vi "运维调试_CODCr.vi"() -> ()   [LabVIEW 2016, in "CODCr库.lvlib"]
uses:
  <vilib>/Utility/miscctls.llb/LVPointTypeDef.ctl
  <vilib>/ptbypt/NI_PtbyPt.lvlib
  <vilib>/Utility/config.llb/NI_LVConfig.lvlib
panel:
  in  "MB通信方式选择":enum16{"串口", "TCP"}(ring)
  in  "释放串口":bool
  in  "打开串口":bool
  in  "加标回收测试":bool
  in  "平行样测试":bool
  in  "定时启动":bool
  out "COM口":string
  in  "空白测试":bool
  in  "隐藏按钮":bool
  in  "写入消解温度时长":bool
  in  "保存KB值":bool
  in  "标样核查":bool
  out "启动时间":timestamp format="%<%Y/%m/%d %H:%M:%S>T"
  out "主循环次数":i32
  out "status":bool
  out "启动测量模式":T1(ring)
  out "曲线斜率B":sgl format="%#_10g"
  out "曲线斜率K":sgl format="%#_10g"
  out "量程上限":sgl
  out "量程下限":sgl
  out "消解时长":u16
  out "消解温度":u16
  out "测量精度":u16
  out "测量结果":sgl
  out "标样参考值":sgl
  out "量程":u16
  out "工作状态":T1(ring)
  out "仪器时间":timestamp format="%<%X\n%x>T"
  out "关键参数区":T2
  out "状态告警区":T3
  out "测量数据区":T4 {"单位" items=["ug/L", "mg/L", "ppm", "mg/m3", "cm", "ppb", "ug/m3", "%", "nmol/mol", "umol/mol", "MPN/L", "MPN/100ml", "ng/m3", "NTU", "无量纲", "ms/cm", "us/cm", "℃", "mV", "万个/L"]}
  out "系统时间":timestamp format="%<%Y/%m/%d %H:%M:%S>T"
  in  "停止":bool
  in  "校时":bool
  in  "标样校准":bool
  in  "空白校准":bool
  in  "零点核查":bool
  in  "跨度核查":bool
  in  "水样测试":bool
  in  "返回":bool
  in  "设置":bool
  # "mg/L"
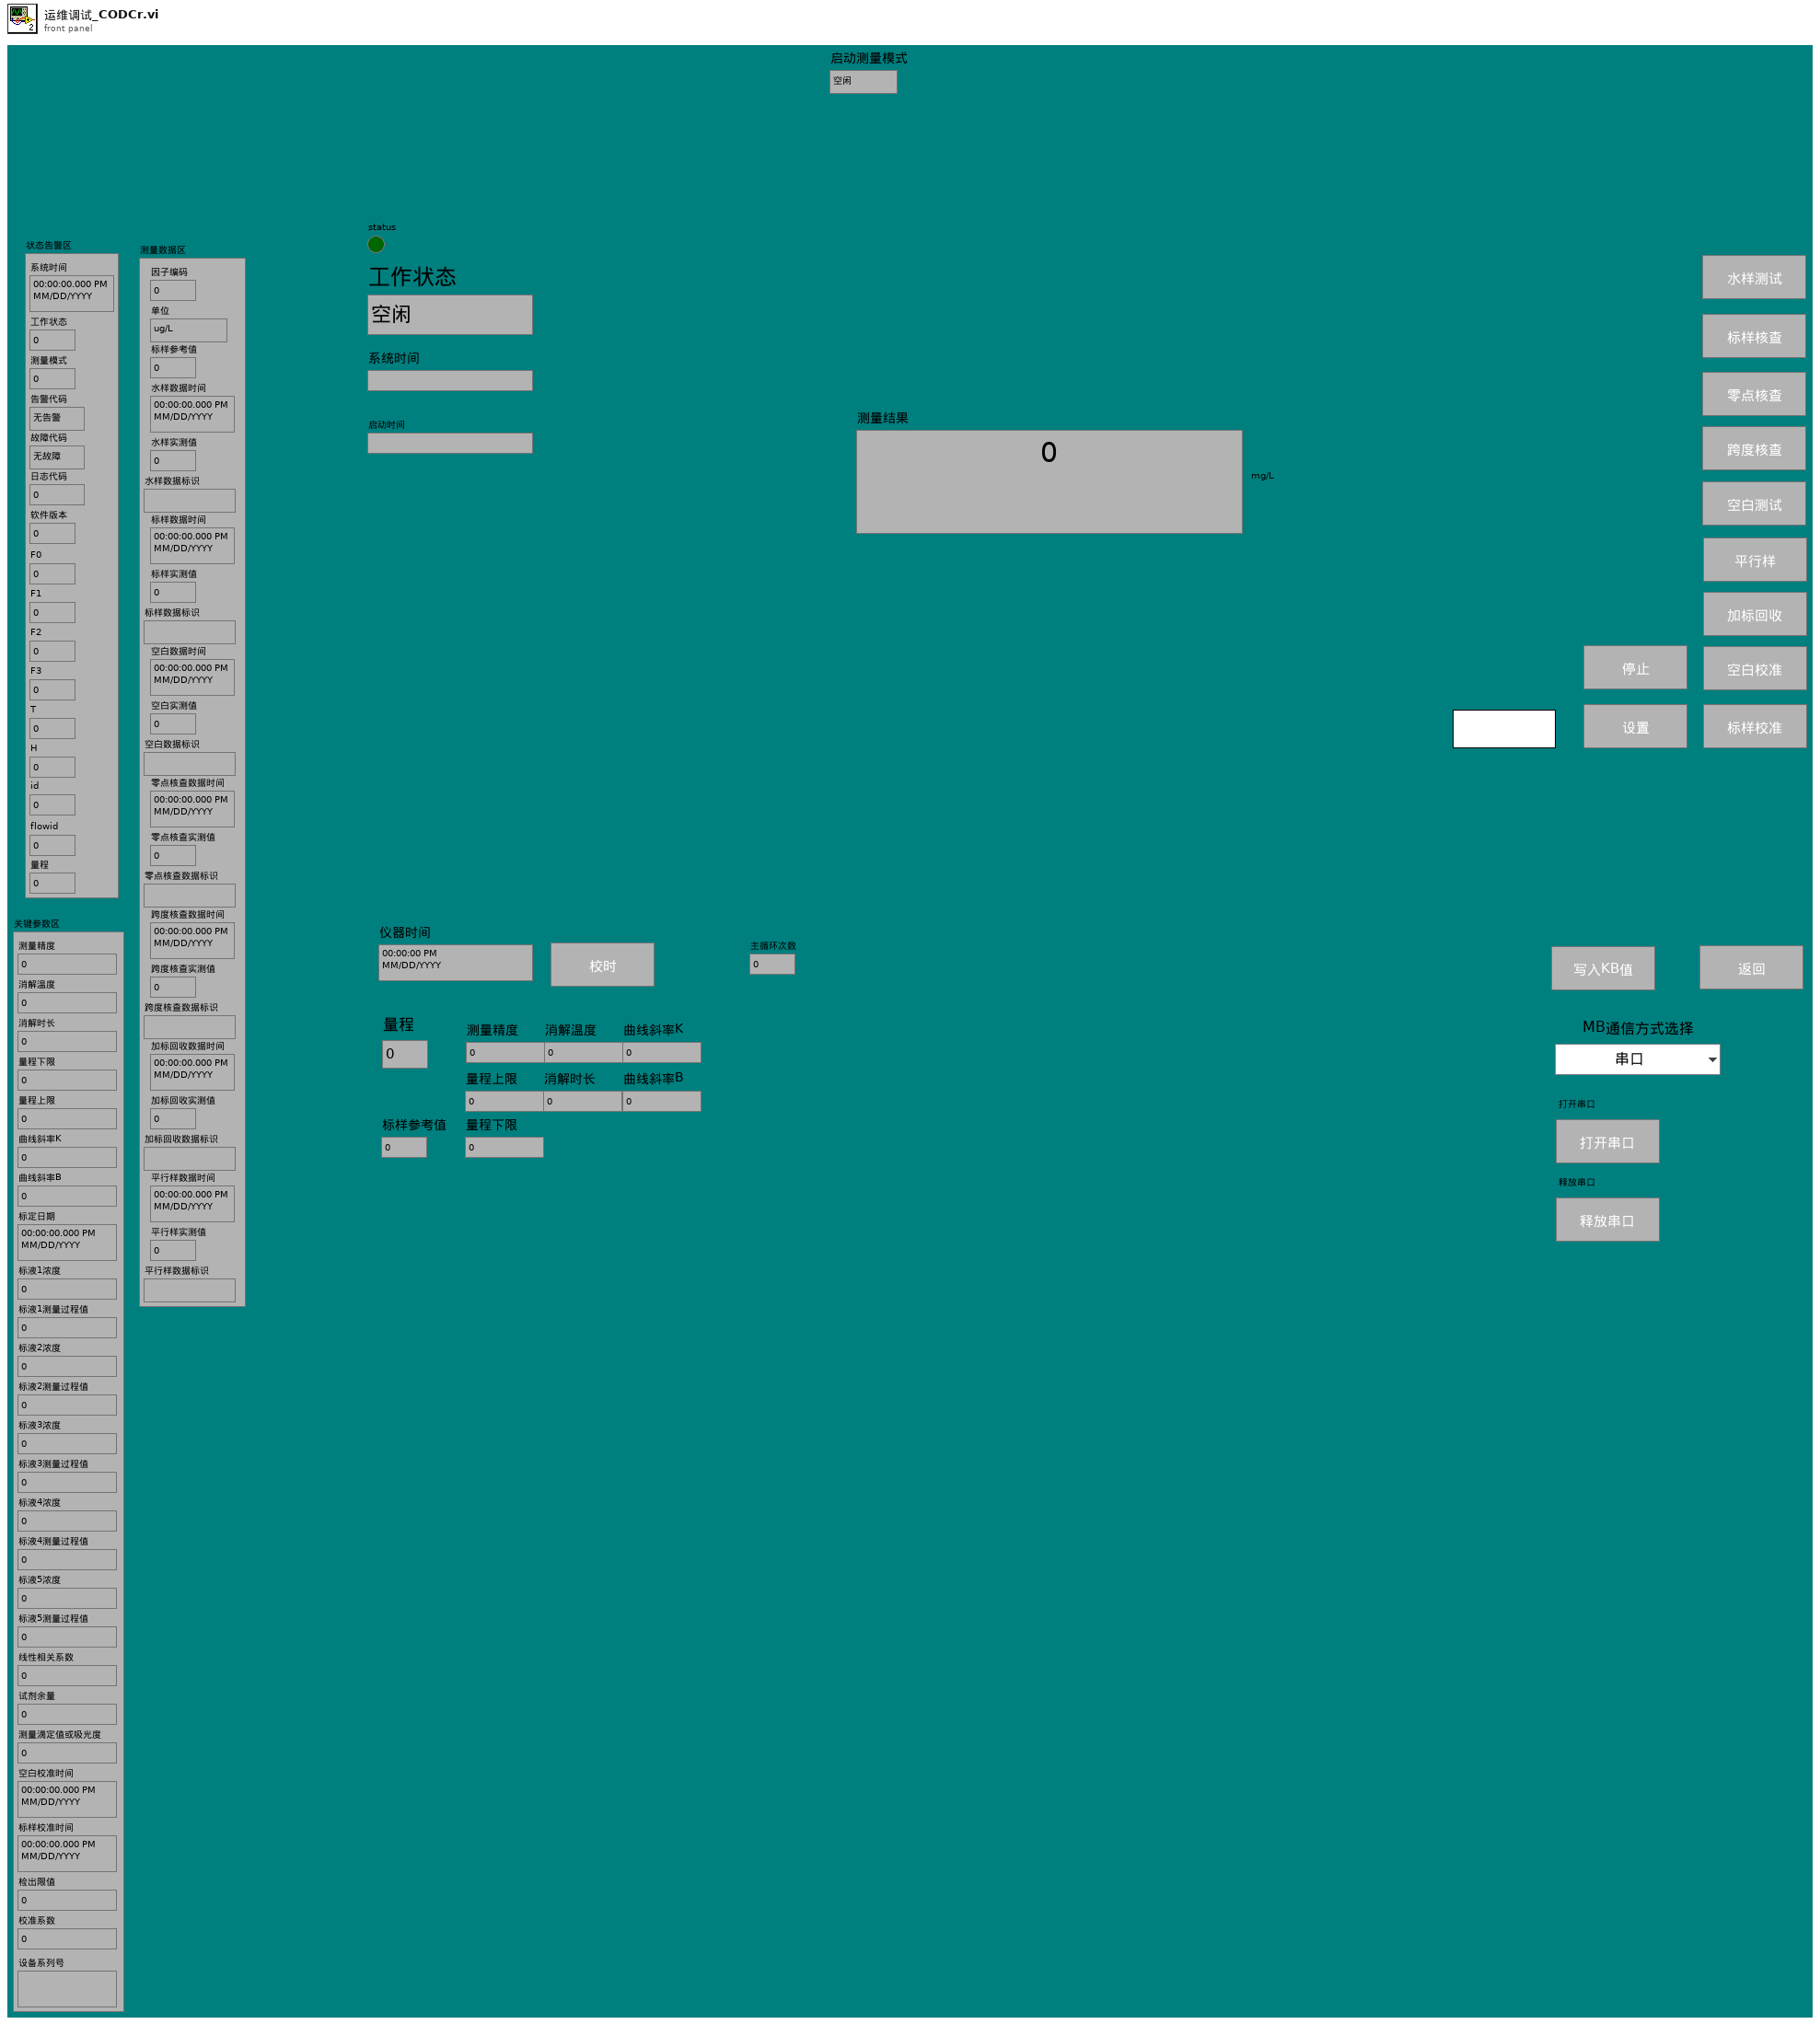
[diagram p1: front panel]
types:
  T1 = enum16{"空闲", "水样测试", "标样核查", "零点核查", "跨度核查", "空白测试", "平行样测试", "加标回收", "空白校准", "标样校准", "初始化（清洗）"}
  T2 = cluster{"测量精度":u16, "消解温度":u16, "消解时长":u16, "量程下限":sgl, "量程上限":sgl, "曲线斜率K":sgl, "曲线斜率B":sgl, "标定日期":timestamp, "标液1浓度":sgl, "标液1测量过程值":sgl, "标液2浓度":sgl, "标液2测量过程值":sgl, "标液3浓度":sgl, "标液3测量过程值":sgl, "标液4浓度":sgl, "标液4测量过程值":sgl, "标液5浓度":sgl, "标液5测量过程值":sgl, "线性相关系数":sgl, "试剂余量":u32, "测量滴定值或吸光度":sgl, "空白校准时间":timestamp, "标样校准时间":timestamp, "检出限值":sgl, "校准系数":sgl, "设备系列号":string}
  T3 = cluster{"系统时间":timestamp, "工作状态":u16, "测量模式":u16, "告警代码":enum16{"无告警", "缺试剂告警", "缺水样告警", "缺蒸馏水告警", "缺标液告警", "仪表漏液告警", "标定异常告警", "超量程告警", "加热异常", "低试剂预警", "超上限告警", "超下限告警", "仪表内部其他异常", "滴定异常告警", "电极异常告警", "量程切换告警", "参数设置告警", "PH电极电位异常", "电导率电极异常", "浊度光度异常", "溶解氧电极异常", "溶解氧光强异常", "温度异常告警", "PH异常告警", "溶解氧异常告警", "电导率异常告警", "浊度异常告警", "叶绿素异常告警", "藻密度异常告警", "蓝绿藻异常告警", "ORP异常告警", "氨氮异常告警", "清洁刷异常告警", "SD卡异常告警", "蓝牙异常告警", "Wifi异常告警", "流程异常告警"}, "故障代码":enum16{"无故障", "电机故障", "温度故障", "通讯故障", "滴定故障"}, "日志代码":u16, "软件版本":u16, "F0":sgl, "F1":sgl, "F2":sgl, "F3":sgl, "T":sgl, "H":sgl, "id":u16, "flowid":u16, "量程":u16}
  T4 = cluster{"因子编码":u32, "单位":u16, "标样参考值":sgl, "水样数据时间":timestamp, "水样实测值":sgl, "水样数据标识":string, "标样数据时间":timestamp, "标样实测值":sgl, "标样数据标识":string, "空白数据时间":timestamp, "空白实测值":sgl, "空白数据标识":string, "零点核查数据时间":timestamp, "零点核查实测值":sgl, "零点核查数据标识":string, "跨度核查数据时间":timestamp, "跨度核查实测值":sgl, "跨度核查数据标识":string, "加标回收数据时间":timestamp, "加标回收实测值":sgl, "加标回收数据标识":string, "平行样数据时间":timestamp, "平行样实测值":sgl, "平行样数据标识":string}
  T5 = cluster{"命令":string, "测量模式":enum16{"水样测量", "标样核查", "零点核查", "跨度核查", "空白测试", "加标回收", "平行样", "校零", "校标"}, "CODCr量程切换":enum32{"H", "L", "AUTO"}}
  T6 = cluster{"测量模式":enum16{"水样测量", "标样核查", "零点核查", "跨度核查", "空白测试", "加标回收", "平行样", "校零", "校标"}}
  T7 = cluster{"仪器测试类型":enum16{"水样测试", "标样核查", "空白测试", "跨度核查"}, "周期设置类型":enum16{"定点启动", "间隔启动"}, "定时功能启用":bool, "定时间隔":dbl, "24H周期设置":bool[]}
  T8 = typedef "LVDateTimeRec.ctl" = cluster{"秒数的小数部分":dbl, "秒":i32, "分":i32, "时":i32, "日":i32, "月":i32, "年":i32, "天数（周）":i32, "天数（年）":i32, "DST":i32}
  T9 = typedef "LVPointTypeDef.ctl" = cluster{"Horizontal":i16, "Vertical":i16}
  T10 = typedef "NI_LVConfig.lvlib/Config Data RefNum.ctl" = refnum<k1>
  T11 = cluster{"运行模式":enum16{"维护模式", "常规模式", "应急模式", "质控模式"}}
  T12 = cluster{"时间标识":timestamp, "监测值":sgl, "单位":u16, "数据标识":string, "因子编码":u32, "标样参考值":sgl, "F0":sgl, "F1":sgl, "F2":sgl, "F3":sgl, "温度":sgl, "湿度":sgl, "量程标识":string}
  T13 = cluster{"时间标识":timestamp, "设备":string, "日志信息":string}
  T14 = cluster{"时间标识":timestamp, "参数":string, "日志信息":string, "流程参数":string}
  T15 = enum16{"无告警", "缺试剂告警", "缺水样告警", "缺蒸馏水告警", "缺标液告警", "仪表漏液告警", "标定异常告警", "超量程告警", "加热异常", "低试剂预警", "超上限告警", "超下限告警", "仪表内部其他异常", "滴定异常告警", "电极异常告警", "量程切换告警", "参数设置告警", "PH电极电位异常", "电导率电极异常", "浊度光度异常", "溶解氧电极异常", "溶解氧光强异常", "温度异常告警", "PH异常告警", "溶解氧异常告警", "电导率异常告警", "浊度异常告警", "叶绿素异常告警", "藻密度异常告警", "蓝绿藻异常告警", "ORP异常告警", "氨氮异常告警", "清洁刷异常告警", "SD卡异常告警", "蓝牙异常告警", "Wifi异常告警", "流程异常告警"}
  T16 = cluster{"时间标识":timestamp, "设备":string, "日志信息":string, "流程参数":string}
  T17 = enum16{"水样测量", "标样核查", "零点核查", "跨度核查", "空白测试", "加标回收", "平行样", "校零", "校标"}
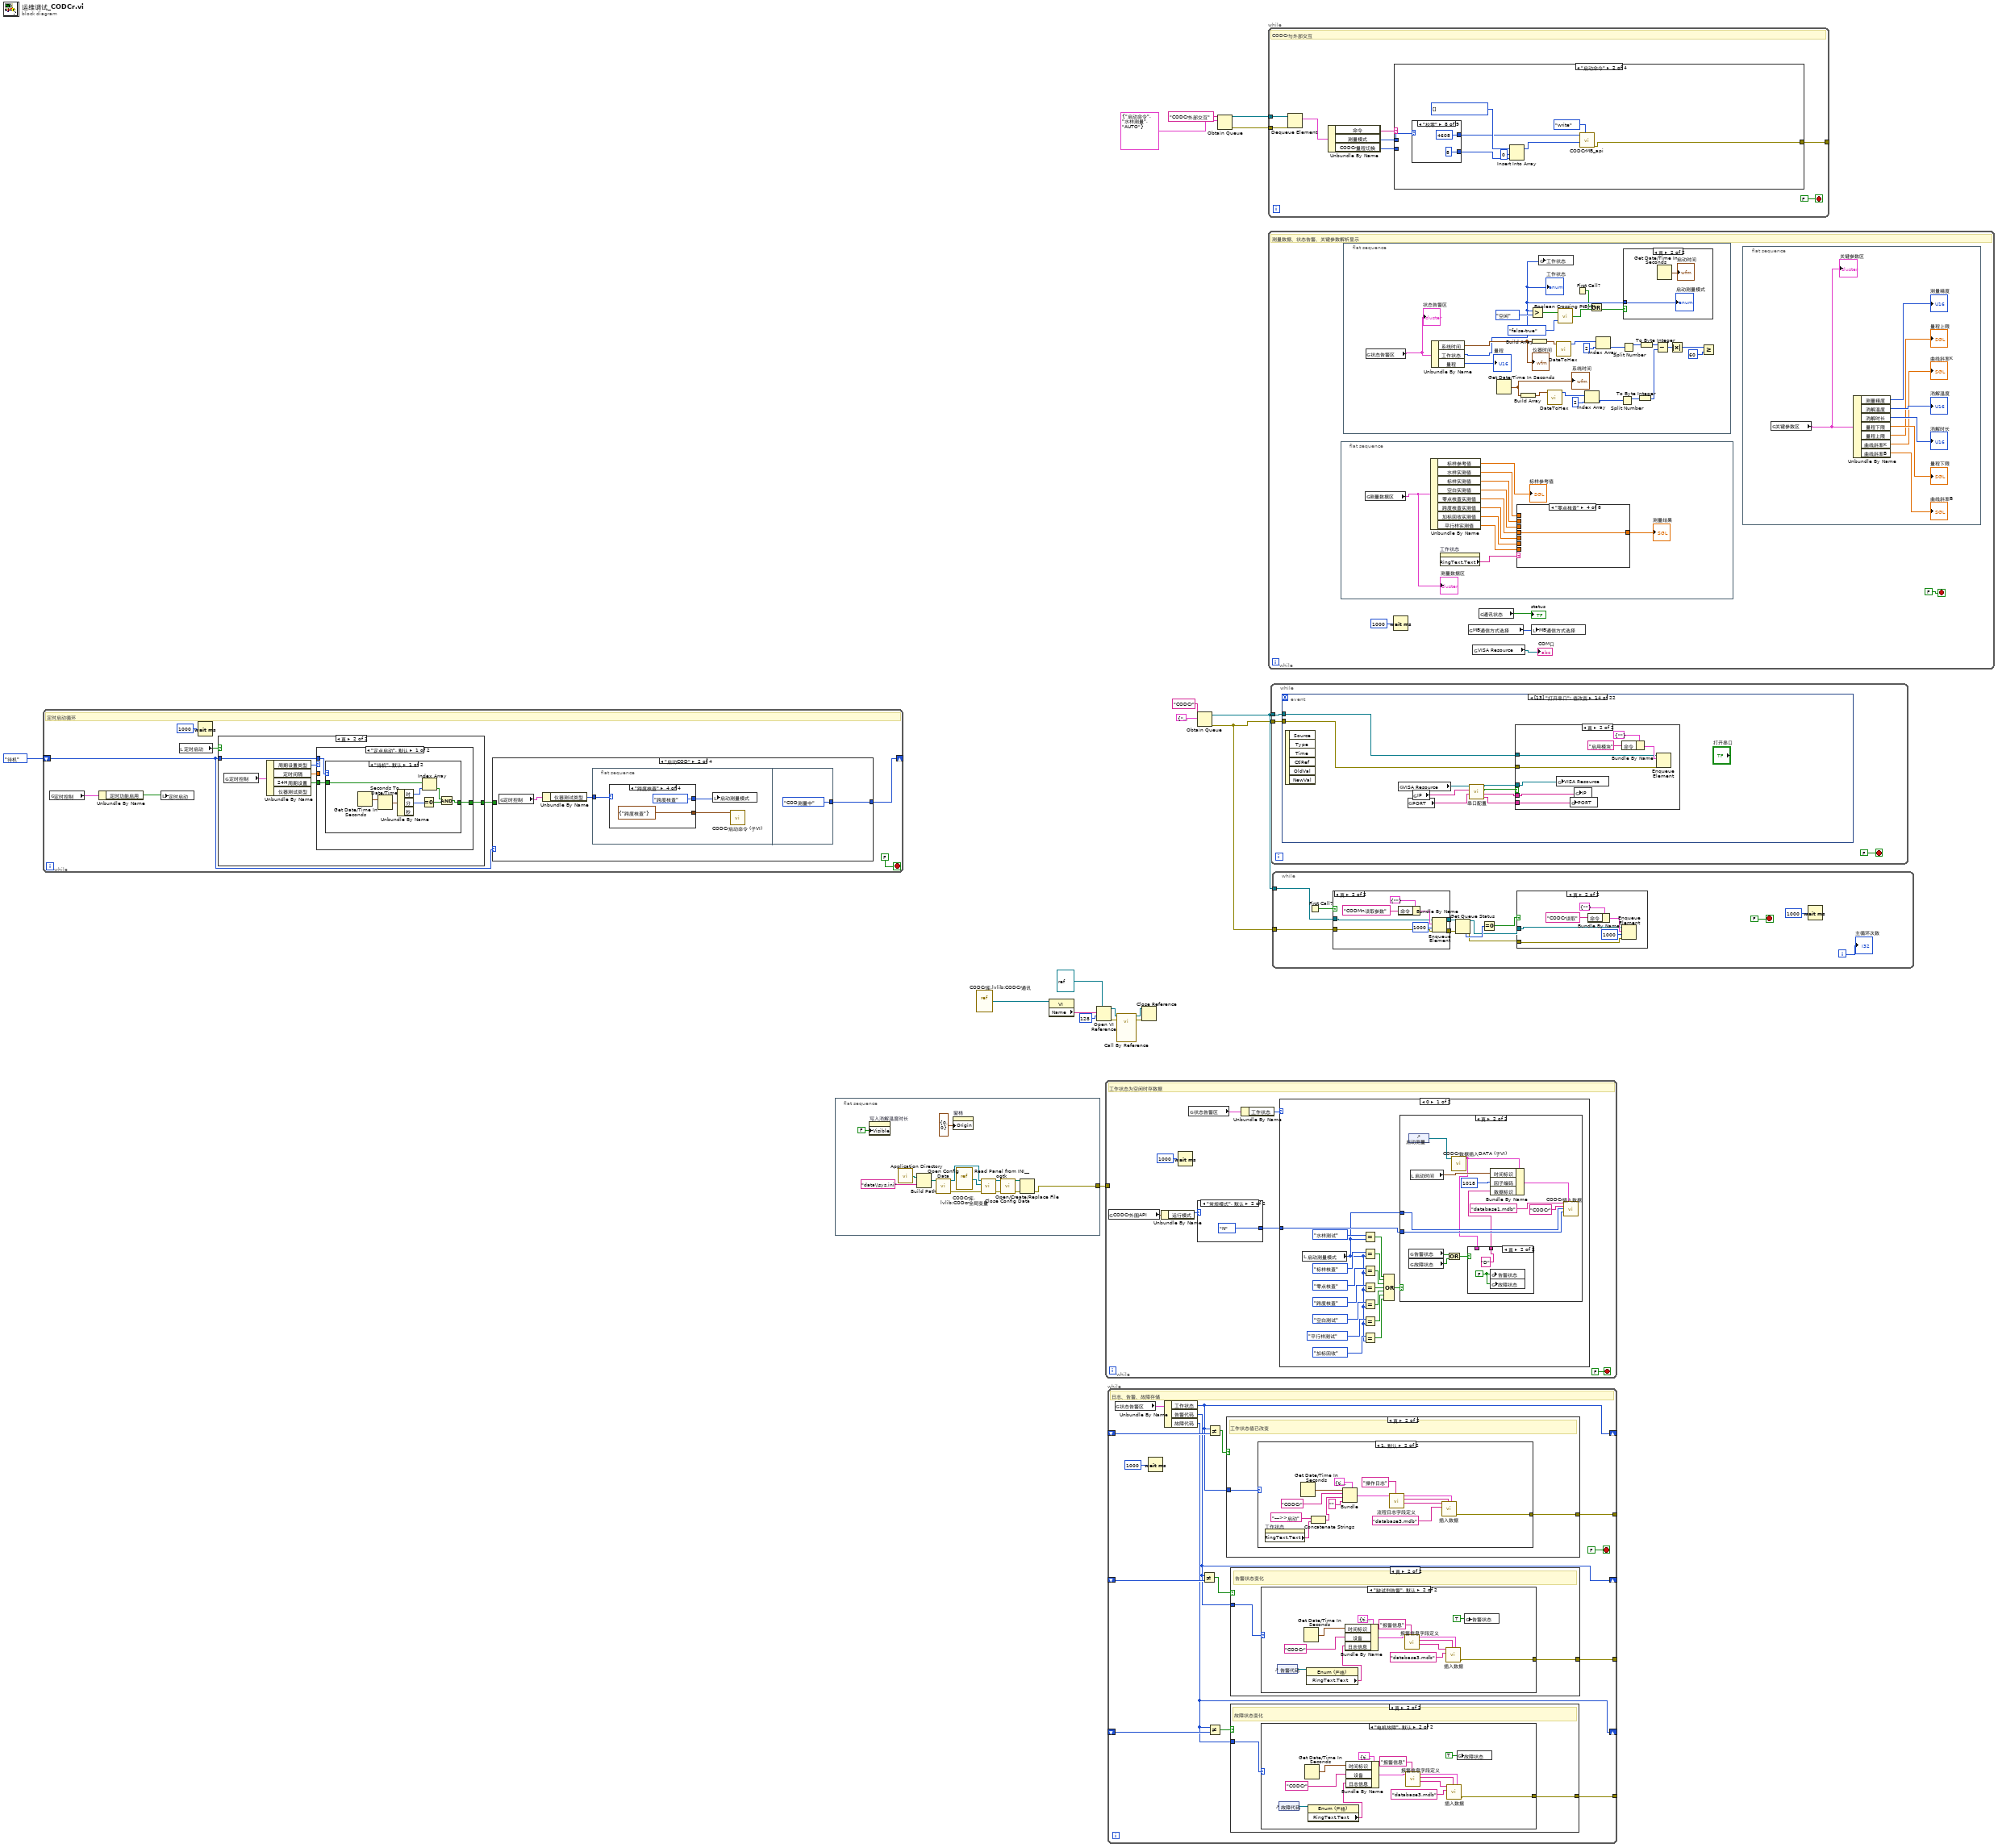
[diagram p0: block diagram]
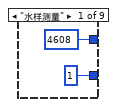
[diagram p5: hidden frame]
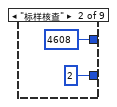
[diagram p6: hidden frame]
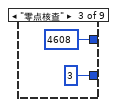
[diagram p7: hidden frame]
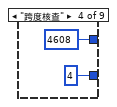
[diagram p8: hidden frame]
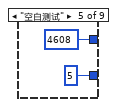
[diagram p9: hidden frame]
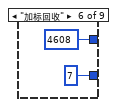
[diagram p10: hidden frame]
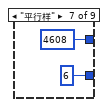
[diagram p11: hidden frame]
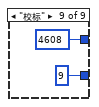
[diagram p12: hidden frame]
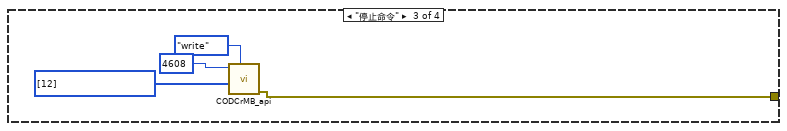
[diagram p13: hidden frame]
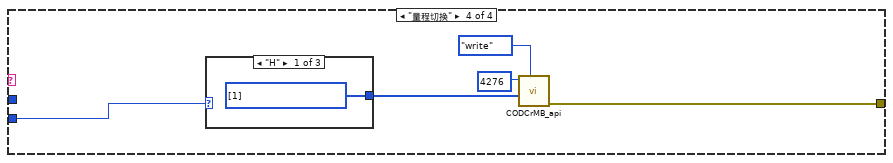
[diagram p14: hidden frame]
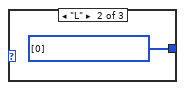
[diagram p15: hidden frame]
diagram:
  n1 = while {
    shift-right: [w24] -> _
    shift-left: enum16{"待机", "启动COD", "COD测量中", "延时"}."待机" -> [w23]
    stop <- FALSE stop-if-true
    # "定时启动循环"
    n2 = global read "CODcr全局变量.vi" "定时控制"() -> (w20:T7)
    n3 = Unbundle By Name(w20) -> ("定时功能启用"=w19:bool)
    n4 = local write "定时启动"(w19) -> ()
    n5 = local read "定时启动"() -> (w21:bool)
    n6 = Wait (ms)(milliseconds to wait=u32 1000 ("等待时间（毫秒）")) -> ()  [unwired: 1 out]
    n7 = case shown="真" w21 {
      tunnel: w23 -> [_ w59]
      tunnel: [_ w58] -> w22
      frame False {
      }
      frame True {
        n8 = global read "CODcr全局变量.vi" "定时控制"() -> (w57:T7)
        n9 = Unbundle By Name(w57) -> ("周期设置类型"=w60:enum16{"定点启动", "间隔启动"}, "定时间隔"=w61:dbl, "24H周期设置"=w62:bool[])  [unwired: 1 out]
        n10 = case shown="\"定点启动\", 默认" w60 {
          tunnel: w61 -> [_ w77]
          tunnel: w62 -> [w65 _]
          tunnel: w59 -> [w63 w80]
          tunnel: [w64 w75] -> w58
          frame "定点启动", Default {
            n11 = case shown="\"待机\", 默认" w63 {
              tunnel: w65 -> [w71 _]
              tunnel: [w66 _] -> w64
              frame "待机", Default {
                n12 = Get Date/Time In Seconds() -> (seconds since 1Jan1904=w73:timestamp)
                n13 = Seconds To Date/Time(time stamp (now)=w73) -> (date time rec=w72:T8)  [unwired: 1 in]
                n14 = Unbundle By Name(w72) -> ("时"=w70:i32, "分"=w69:i32)  [unwired: 1 out]
                n15 = Equal To 0?(x=w69) -> (x = 0?=w67:bool)
                n16 = Index Array(array=w71, index=w70) -> (element=w68:bool)
                n17 = Compound Arithmetic op=AND ("复合运算")(w68, w67) -> (w66:bool)
              }
              frame "启动COD" {
              }
            }
          }
          frame "间隔启动" {
            n18 = Multiply(x=w77, y=60.0) -> (x*y=w74:dbl)
            n19 = feedback #1(w74) -> (w79:dbl)
            n20 = case shown="\"待机\"" w80 {
              tunnel: w79 -> [_ w82]
              tunnel: [_ w81] -> w78
              frame Default {
              }
              frame "待机" {
                n21 = Increment(x=w82) -> (x+1=w81:dbl)
              }
            }
            n22 = feedback-in #1(w78) -> ()
            n23 = Greater Or Equal?(x=w78, y=w74) -> (x >= y?=w75:bool)
          }
        }
      }
    }
    n24 = case shown="\"启动COD\"" w23 {
      tunnel: [w27 w33 w47 enum16{"待机", "启动COD", "COD测量中", "延时"}."待机"] -> w24
      tunnel: w22 -> [w30 _ _ _]
      frame "待机", Default {
        n25 = Select(t=enum16{"待机", "启动COD", "COD测量中", "延时"}."启动COD", s=w30, f=enum16{"待机", "启动COD", "COD测量中", "延时"}."待机") -> (s? t:f=w27:enum16{"待机", "启动COD", "COD测量中", "延时"})
      }
      frame "启动COD" {
        n26 = global read "CODcr全局变量.vi" "定时控制"() -> (w31:T7)
        n27 = Unbundle By Name(w31) -> ("仪器测试类型"=w32:enum16{"水样测试", "标样核查", "空白测试", "跨度核查"})
        n28 = flat-sequence {
          tunnel: w32 -> [w36]
          tunnel: [enum16{"待机", "启动COD", "COD测量中", "延时"}."COD测量中"] -> w33
          frame #0 {
            n29 = case shown="\"跨度核查\"" w36 {
              tunnel: [T6 {"测量模式"=enum."水样测量"} ("启动测量模式") T6 {"测量模式"=enum."标样核查"} ("启动测量模式") T6 {"测量模式"=enum."空白测试"} ("启动测量模式") T6 {"测量模式"=enum."跨度核查"} ("启动测量模式")] -> w35
              tunnel: [T1."水样测试" ("启动测量模式") T1."标样核查" ("启动测量模式") T1."空白测试" ("启动测量模式") T1."跨度核查" ("启动测量模式")] -> w34
              frame "水样测试", Default {
              }
              frame "标样核查" {
              }
              frame "空白测试" {
              }
              frame "跨度核查" {
              }
            }
            n30 = local write "启动测量模式"(w34) -> ()
            n31 = call "CODCr启动命令 (子VI).vi"("启动测量模式"=w35) -> ()  [unwired: 11 in]
          }
          frame #1 {
          }
        }
      }
      frame "COD测量中" {
        n32 = flat-sequence {
          tunnel: [w51] -> w46
          tunnel: [w55] -> w47
          tunnel: w46 -> [w55]
          frame #0 {
            n33 = local read "状态告警区"() -> (w50:T3)
            n34 = Unbundle By Name(w50) -> ("工作状态"=w49:u16)
            n35 = Equal To 0?(x=w49) -> (x = 0?=w48:bool)
            n36 = Select(t=enum16{"待机", "启动COD", "COD测量中", "延时"}."延时", s=w48, f=enum16{"待机", "启动COD", "COD测量中", "延时"}."COD测量中") -> (s? t:f=w51:enum16{"待机", "启动COD", "COD测量中", "延时"})
          }
          frame #1 {
            n37 = Wait (ms)(milliseconds to wait=u32 5000 ("等待时间（毫秒）")) -> ()  [unwired: 1 out]
          }
        }
      }
      frame "延时" {
      }
    }
  }
  n38 = flat-sequence {
    tunnel: [w83] -> w17
    frame #0 {
      n39 = property on="写入消解温度时长" class="Bool"("Visible"=FALSE ("可见")) -> ()  [unwired: 2 in, 2 out]
      n40 = call <vilib>:"Application Directory.vi"() -> ("Application Directory"=w93:path)
      n41 = Build Path(base path=w93, name or relative path="data\\sys.ini" ("名称或相对路径")) -> (appended path=w91:path)
      n42 = call <vilib>:"Open Config Data.vi"("configuration file path"=w91) -> ("error out"=w87:errorcluster, "refnum"=w90:T10)  [unwired: 8 in, 1 out]
      n43 = property on="窗格" class="Pane"("Origin"=T9 {"Horizontal"=0, "Vertical"=0} ("原点")) -> ()  [unwired: 2 in, 2 out]
      n44 = vi-ref "CODCr库.lvlib:CODcr全局变量.vi"() -> (w89:refnum<vi>)
      n45 = call <userlib>:"Read Panel from INI__ogtk.vi"("error in (no error)"=w87, "VI ref"=w89, "refnum"=w90) -> ("error out"=w86:errorcluster, "refnum out"=w88:T10)  [unwired: 7 in]
      n46 = call <vilib>:"Close Config Data.vi"("error in (no error)"=w86, "refnum"=w88) -> ("error out"=w85:errorcluster, "file path"=w84:path)  [unwired: 8 in]
      n47 = Open/Create/Replace File(file path (use dialog)=w84, error in=w85) -> (error out=w83:errorcluster)  [unwired: 4 in, 2 out]
    }
  }
  n48 = vi-ref "CODCr库.lvlib:CODCr通讯.vi"() -> (w9:refnum<vi>)
  n49 = property class="VI"(reference=w9) -> ("Name"=w10:string)  [unwired: 1 in, 2 out]
  n50 = Open VI Reference(type specifier VI Refnum (for type only)=refnum<vi> refnum, vi path=w10, options=128 ("选项")) -> (vi reference=w12:refnum<vi>, error out=w14:errorcluster)  [unwired: 3 in]
  n51 = while "While循环" {
    tunnel: w17 -> [_]
    stop <- FALSE stop-if-true
    # "工作状态为空闲时存数据"
    n52 = global read "CODCr外部API.vi" "CODCr外围API"() -> (w98:T11)
    n53 = Unbundle By Name(w98) -> ("运行模式"=w97:enum16{"维护模式", "常规模式", "应急模式", "质控模式"})
    n54 = Wait (ms)(milliseconds to wait=u32 1000 ("等待时间（毫秒）")) -> ()  [unwired: 1 out]
    n55 = global read "CODcr全局变量.vi" "状态告警区"() -> (w96:T3)
    n56 = case shown="\"常规模式\", 默认" w97 {
      tunnel: [enum16{"N", "M"}."M" ("数据类型") enum16{"N", "M"}."N" ("数据类型")] -> w99
      frame "维护模式" {
      }
      frame "常规模式", Default {
      }
    }
    n57 = Unbundle By Name(w96) -> ("工作状态"=w100:u16)
    n58 = case shown="0" w100 {
      tunnel: w99 -> [w121 _]
      frame 0 {
        n59 = local read "启动测量模式"() -> (w113:T1)
        n60 = Equal?(x=T1."水样测试" ("启动测量模式"), y=w113) -> (x = y?=w112:bool)
        n61 = Equal?(x=T1."标样核查" ("启动测量模式"), y=w113) -> (x = y?=w111:bool)
        n62 = Equal?(x=T1."零点核查" ("启动测量模式"), y=w113) -> (x = y?=w110:bool)
        n63 = Equal?(x=T1."跨度核查" ("启动测量模式"), y=w113) -> (x = y?=w109:bool)
        n64 = Equal?(x=T1."空白测试" ("启动测量模式"), y=w113) -> (x = y?=w108:bool)
        n65 = Equal?(x=T1."平行样测试" ("启动测量模式"), y=w113) -> (x = y?=w107:bool)
        n66 = Equal?(x=T1."加标回收" ("启动测量模式"), y=w113) -> (x = y?=w106:bool)
        n67 = Compound Arithmetic op=OR(w112, w111, w110, w109, w108, w107, w106) -> (w105:bool)
        n68 = case shown="真" w105 {
          tunnel: w113 -> [_ w129]
          tunnel: w121 -> [_ w128]
          frame False {
          }
          frame True {
            n69 = control-ref of="启动测量模式"() -> (w133:refnum<vi>)
            n70 = global read "CODcr全局变量.vi" "告警状态"() -> (w126:bool)
            n71 = global read "CODcr全局变量.vi" "故障状态"() -> (w125:bool)
            n72 = local read "启动时间"() -> (w134:timestamp)
            n73 = Or(x=w126, y=w125) -> (x .or. y?=w124:bool)
            n74 = call "CODCr数据插入DATA (子VI).vi"("Enum输入"=w133) -> ("data"=w123:T12)  [unwired: 10 in]
            n75 = case shown="真" w124 {
              tunnel: w123 -> [w136 _]
              tunnel: [w135 "D" ("table")] -> w122
              frame False {
                n76 = Unbundle By Name(w136) -> ("数据标识"=w135:string)
              }
              frame True {
                w137 = FALSE ("告警状态")
                n77 = global write "CODcr全局变量.vi" "告警状态"(w137) -> ()
                n78 = global write "CODcr全局变量.vi" "故障状态"(w137) -> ()
              }
            }
            n79 = Bundle By Name(cluster=w123, "时间标识"=w134, "因子编码"=u32 1018, "数据标识"=w122) -> (w132:T12)
            n80 = call "CODCr插入数据.vi"("database"="database1.mdb", "data"=w132, "table"="CODCr", "测量模式"=w129, "数据类型"=w128) -> ()  [unwired: 10 in, 1 out]
          }
        }
      }
      frame 1, Default {
      }
    }
  }
  n81 = while {
    shift-right: [w149] -> _
    shift-left: _ -> [w151]
    tunnel: [w148] -> _
    shift-right: [w144] -> _
    shift-left: _ -> [w145]
    shift-right: [w140] -> _
    shift-left: _ -> [w142]
    tunnel: [w141] -> _
    tunnel: [w139] -> _
    stop <- FALSE stop-if-true
    # "日志、告警、故障存储"
    n82 = global read "CODcr全局变量.vi" "状态告警区"() -> (w147:T3)
    n83 = Wait (ms)(milliseconds to wait=u32 1000 ("等待时间（毫秒）")) -> ()  [unwired: 1 out]
    n84 = Unbundle By Name(w147) -> ("工作状态"=w149:u16, "告警代码"=w144:T15, "故障代码"=w140:enum16{"无故障", "电机故障", "温度故障", "通讯故障", "滴定故障"})
    n85 = Not Equal?(x=w144, y=w145) -> (x != y?=w146:bool)
    n86 = Not Equal?(x=w149, y=w151) -> (x != y?=w150:bool)
    n87 = Not Equal?(x=w140, y=w142) -> (x != y?=w143:bool)
    n88 = case shown="真" w150 {
      tunnel: w149 -> [_ w185]
      tunnel: [_ w184] -> w148
      frame False {
      }
      frame True {
        # "工作状态值已改变"
        n89 = case shown="1, 默认" w185 {
          tunnel: [w186 w201] -> w184
          frame 0 {
            n90 = Get Date/Time In Seconds() -> (seconds since 1Jan1904=w193:timestamp)
            n91 = Bundle(cluster=T14 {"时间标识"=timestamp(0 s since 1904-01-01), "参数"="", "日志信息"="", "流程参数"=""} ("data in"), "时间标识"=w193, "参数"="CODCr" ("table输入"), "日志信息"="--->>结束", "流程参数"="" ("table输入")) -> (w187:T14)
            n92 = call "流程日志字段定义.vi"("table输入"="操作日志", "data in"=w187) -> ("table输出"=w191:string, "columns"=w189:string[], "data out"=w188:T16)  [unwired: 7 in]
            n93 = call "插入数据.vi"("data"=w188, "columns"=w189, "database"="database3.mdb", "table"=w191) -> ("error out"=w186:errorcluster)  [unwired: 7 in]
          }
          frame 1, Default {
            n94 = property on="工作状态" class="Enum (严格)"() -> ("RingText.Text"=w198:string)  [unwired: 2 in, 2 out]
            n95 = Get Date/Time In Seconds() -> (seconds since 1Jan1904=w208:timestamp)
            n96 = Concatenate Strings("--->>启动" ("日志信息"), w198) -> (w199:string)
            n97 = Bundle(cluster=T14 {"时间标识"=timestamp(0 s since 1904-01-01), "参数"="", "日志信息"="", "流程参数"=""} ("data in"), "时间标识"=w208, "参数"="CODCr" ("table输入"), "日志信息"=w199, "流程参数"="" ("table输入")) -> (w207:T14)
            n98 = call "流程日志字段定义.vi"("table输入"="操作日志", "data in"=w207) -> ("table输出"=w205:string, "columns"=w203:string[], "data out"=w202:T16)  [unwired: 7 in]
            n99 = call "插入数据.vi"("data"=w202, "columns"=w203, "database"="database3.mdb", "table"=w205) -> ("error out"=w201:errorcluster)  [unwired: 7 in]
          }
        }
      }
    }
    n100 = case shown="真" w143 {
      tunnel: w140 -> [_ w155]
      tunnel: [_ w154] -> w139
      frame False {
      }
      frame True {
        # "故障状态变化"
        n101 = case shown="\"电机故障\", 默认" w155 {
          tunnel: [_ w157] -> w154
          frame "无故障" {
            # "无告警"
          }
          frame "电机故障", Default {
            n102 = control-ref of="故障代码"() -> (w167:refnum<vi>)
            n103 = Get Date/Time In Seconds() -> (seconds since 1Jan1904=w165:timestamp)
            n104 = property class="Enum (严格)"(reference=w167) -> ("RingText.Text"=w168:string)  [unwired: 1 in, 2 out]
            n105 = Bundle By Name(cluster=T13 {"时间标识"=timestamp(0 s since 1904-01-01), "设备"="", "日志信息"=""} ("data in"), "时间标识"=w165, "设备"="CODCr" ("table输入"), "日志信息"=w168) -> (w164:T13)
            n106 = call "报警信息字段定义.vi"("table输入"="报警信息", "data in"=w164) -> ("table输出"=w159:string, "columns"=w158:string[], "data out"=w161:T13)  [unwired: 7 in]
            n107 = call "插入数据.vi"("data"=w161, "columns"=w158, "database"="database3.mdb", "table"=w159) -> ("error out"=w157:errorcluster)  [unwired: 7 in]
            n108 = global write "CODcr全局变量.vi" "故障状态"(TRUE ("告警状态")) -> ()
          }
        }
      }
    }
    n109 = case shown="真" w146 {
      tunnel: w144 -> [_ w170]
      tunnel: [_ w169] -> w141
      frame False {
      }
      frame True {
        # "告警状态变化"
        n110 = case shown="\"缺试剂告警\", 默认" w170 {
          tunnel: [_ w176] -> w169
          frame "无告警" {
            # "无告警"
          }
          frame "缺试剂告警", Default {
            n111 = control-ref of="告警代码"() -> (w173:refnum<vi>)
            n112 = Get Date/Time In Seconds() -> (seconds since 1Jan1904=w175:timestamp)
            n113 = property class="Enum (严格)"(reference=w173) -> ("RingText.Text"=w172:string)  [unwired: 1 in, 2 out]
            n114 = Bundle By Name(cluster=T13 {"时间标识"=timestamp(0 s since 1904-01-01), "设备"="", "日志信息"=""} ("data in"), "时间标识"=w175, "设备"="CODCr" ("table输入"), "日志信息"=w172) -> (w177:T13)
            n115 = call "报警信息字段定义.vi"("table输入"="报警信息", "data in"=w177) -> ("table输出"=w182:string, "columns"=w183:string[], "data out"=w180:T13)  [unwired: 7 in]
            n116 = call "插入数据.vi"("data"=w180, "columns"=w183, "database"="database3.mdb", "table"=w182) -> ("error out"=w176:errorcluster)  [unwired: 7 in]
            n117 = global write "CODcr全局变量.vi" "告警状态"(TRUE ("告警状态")) -> ()
          }
        }
      }
    }
  }
  n118 = call-by-ref "?"(reference=w12, error in=w14) -> (reference out=w16:refnum<vi>, error out=w15:errorcluster)  [unwired: 12 in]
  n119 = Close Reference(reference=w16, error in (no error)=w15) -> ()  [unwired: 1 out]
  n120 = Obtain Queue(name (unnamed)="CODCr" ("名称（未命名）"), element data type=cluster{"命令":string} {"命令"="启用模块"} ("元素")) -> (queue out=w2:refnum<queue>, error out=w1:errorcluster)  [unwired: 3 in, 1 out]
  n121 = Obtain Queue(name (unnamed)="CODCr外部交互" ("名称（未命名）"), element data type=T5 {"命令"="启动命令", "测量模式"=enum."水样测量", "CODCr量程切换"=enum."AUTO"} ("元素")) -> (queue out=w4:refnum<queue>, error out=w3:errorcluster)  [unwired: 3 in, 1 out]
  n122 = while {
    tunnel: w4 -> [w217]
    tunnel: w3 -> [w216]
    tunnel: [w212] -> _
    stop <- FALSE stop-if-true
    # "CODCr与外部交互"
    n123 = Dequeue Element(queue=w217, error in (no error)=w216) -> (element=w218:T5)  [unwired: 1 in, 3 out]
    n124 = Unbundle By Name(w218) -> ("命令"=w215:string, "测量模式"=w214:T17, "CODCr量程切换"=w213:enum32{"H", "L", "AUTO"})
    n125 = case shown="\"启动命令\"" w215 {
      tunnel: w214 -> [_ w221 _ _]
      tunnel: w213 -> [_ _ _ w251]
      tunnel: [_ w220 w246 w250] -> w212
      frame "假", Default {
      }
      frame "启动命令" {
        n126 = case shown="\"校零\"" w221 {
          tunnel: [u16 4608 ("address") u16 4608 ("address") u16 4608 ("address") u16 4608 ("address") u16 4608 ("address") u16 4608 ("address") u16 4608 ("address") u16 4608 ("address") u16 4608 ("address")] -> w223
          tunnel: [u16 1 ("address") u16 2 ("address") u16 3 ("address") u16 4 ("address") u16 5 ("address") u16 7 ("address") u16 6 ("address") u16 8 ("address") u16 9 ("address")] -> w227
          frame "水样测量" {
          }
          frame "标样核查" {
          }
          frame "零点核查" {
          }
          frame "跨度核查" {
          }
          frame "空白测试" {
          }
          frame "加标回收" {
          }
          frame "平行样" {
          }
          frame "校零" {
          }
          frame "校标" {
          }
        }
        n127 = Insert Into Array(array=u16[] [] ("values"), index=0 ("索引"), new element=w227) -> (w222:u16[])
        n128 = call "CODCrMB_api.vi"("STEP"=enum16{"open", "read", "write", "close"}."write", "values"=w222, "starting address"=w223) -> ("error out"=w220:errorcluster)  [unwired: 6 in, 2 out]
      }
      frame "停止命令" {
        n129 = call "CODCrMB_api.vi"("STEP"=enum16{"open", "read", "write", "close"}."write", "values"=u16[] [12], "starting address"=u16 4608) -> ("error out"=w246:errorcluster)  [unwired: 6 in, 2 out]
      }
      frame "量程切换" {
        n130 = case shown="\"H\"" w251 {
          tunnel: [u16[] [1] ("values") u16[] [0] ("values") _] -> w254
          frame "H" {
          }
          frame "L" {
          }
          frame "AUTO", Default {
          }
        }
        n131 = call "CODCrMB_api.vi"("STEP"=enum16{"open", "read", "write", "close"}."write", "values"=w254, "starting address"=u16 4276) -> ("error out"=w250:errorcluster)  [unwired: 6 in, 2 out]
      }
    }
  }
  n132 = while {
    stop <- FALSE stop-if-true
    # "测量数据、状态告警、关键参数解析显示"
    n133 = flat-sequence {
      frame #0 {
        n134 = global read "CODcr全局变量.vi" "测量数据区"() -> (w298:T4)
        "测量数据区" <- w298
        n135 = Unbundle By Name(w298) -> ("标样参考值"=→"标样参考值":sgl, "水样实测值"=w306:sgl, "标样实测值"=w304:sgl, "空白实测值"=w301:sgl, "零点核查实测值"=w303:sgl, "跨度核查实测值"=w302:sgl, "加标回收实测值"=w299:sgl, "平行样实测值"=w300:sgl)
        n136 = property on="工作状态" class="Enum (严格)"() -> ("RingText.Text"=w307:string)  [unwired: 2 in, 2 out]
        n137 = case shown="\"零点核查\"" w307 {
          tunnel: w306 -> [_ w310 _ _ _ _ _ _]
          tunnel: [w309 w310 w311 w312 w313 w314 w315 w316] -> w305
          tunnel: w304 -> [_ _ w311 _ _ _ _ _]
          tunnel: w303 -> [_ _ _ w312 _ _ _ _]
          tunnel: w302 -> [_ _ _ _ w313 _ _ _]
          tunnel: w301 -> [_ _ _ _ _ w314 _ _]
          tunnel: w300 -> [_ _ _ _ _ _ w315 _]
          tunnel: w299 -> [_ _ _ _ _ _ _ w316]
          frame "空闲", Default {
            n138 = local read "测量结果"() -> (w309:sgl)
          }
          frame "水样测试" {
          }
          frame "标样核查" {
          }
          frame "零点核查" {
          }
          frame "跨度核查" {
          }
          frame "空白测试" {
          }
          frame "平行样测试" {
          }
          frame "加标回收" {
          }
        }
        "测量结果" <- w305
      }
    }
    n139 = flat-sequence {
      frame #0 {
        n140 = global read "CODcr全局变量.vi" "状态告警区"() -> (w270:T3)
        "状态告警区" <- w270
        n141 = Unbundle By Name(w270) -> ("系统时间"=w282:timestamp, "工作状态"=w273:u16, "量程"=→"量程":u16)
        "仪器时间" <- w282
        "工作状态" <- w273
        n142 = Get Date/Time In Seconds() -> (seconds since 1Jan1904=w283:timestamp)
        "系统时间" <- w283
        n143 = Build Array(w283) -> (w277:timestamp[])
        n144 = Greater?(x=w273, y=T1."空闲") -> (0:w281:bool)
        n145 = Build Array(w282) -> (w276:timestamp[])
        n146 = global write "CODcr全局变量.vi" "工作状态"(w273) -> ()
        n147 = call "DateToHex.vi"("DATE"=w277) -> ("数组"=w274:u16[])  [unwired: 10 in]
        n148 = call "DateToHex.vi"("DATE"=w276) -> ("数组"=w275:u16[])  [unwired: 10 in]
        n149 = call <vilib>:"Boolean Crossing PtByPt.vi"("direction"=enum16{"either", "false-true", "true-false"}."false-true", "input"=w281) -> ("crossing"=w280:bool)  [unwired: 1 in]
        n150 = First Call?() -> (First Call?: T/F=w271:bool)
        n151 = Index Array(array=w274, index=2 ("索引")) -> (element=w285:u16)
        n152 = Or(x=w271, y=w280) -> (x .or. y?=w272:bool)
        n153 = Index Array(array=w275, index=2 ("索引")) -> (element=w286:u16)
        n154 = Split Number(x=w285) -> (hi(x)=w288:u8)  [unwired: 1 out]
        n155 = Split Number(x=w286) -> (hi(x)=w291:u8)  [unwired: 1 out]
        n156 = case shown="真" w272 {
          tunnel: w273 -> [_ w296]
          frame False {
          }
          frame True {
            n157 = Get Date/Time In Seconds() -> (seconds since 1Jan1904=→"启动时间":timestamp)
            "启动测量模式" <- w296
          }
        }
        n158 = To Byte Integer(number=w288) -> (8bit integer=w289:i8)
        n159 = To Byte Integer(number=w291) -> (8bit integer=w292:i8)
        n160 = Subtract(x=w292, y=w289) -> (x-y=w290:i8)
        n161 = Absolute Value(x=w290) -> (abs(x)=w293:i8)
        n162 = Greater Or Equal?(x=w293, y=i8 60) -> ()  [unwired: 1 out]
      }
    }
    n163 = Wait (ms)(milliseconds to wait=u32 1000 ("等待时间（毫秒）")) -> ()  [unwired: 1 out]
    n164 = global read "CODcr全局变量.vi" "MB通信方式选择"() -> (w258:enum16{"串口", "TCP"})
    n165 = global read "CODcr全局变量.vi" "VISA Resource"() -> (→"COM口":refnum<visa-resource-name>)
    n166 = global read "CODcr全局变量.vi" "通讯状态"() -> (→"status":bool)
    n167 = local write "MB通信方式选择"(w258) -> ()
    n168 = flat-sequence {
      frame #0 {
        n169 = global read "CODcr全局变量.vi" "关键参数区"() -> (w262:T2)
        "关键参数区" <- w262
        n170 = Unbundle By Name(w262) -> ("测量精度"=→"测量精度":u16, "消解温度"=→"消解温度":u16, "消解时长"=→"消解时长":u16, "量程下限"=→"量程下限":sgl, "量程上限"=→"量程上限":sgl, "曲线斜率K"=→"曲线斜率K":sgl, "曲线斜率B"=→"曲线斜率B":sgl)
      }
    }
  }
  n171 = while {
    tunnel: w2 -> [w318]
    tunnel: w1 -> [w317]
    stop <- FALSE stop-if-true
    n172 = event shown="[13] \"打开串口\": 值改变" {
      selector: _ -> [_ _ _ _ _ _ _ _ _ _ _ _ _ _ _ _ _ _ _ _ _ _]
      dyn-events: _ -> [_ _ _ _ _ _ _ _ _ _ _ _ _ _ _ _ _ _ _ _ _ _]
      timeout: _ -> [_ _ _ _ _ _ _ _ _ _ _ _ _ _ _ _ _ _ _ _ _ _]
      tunnel: w318 -> [_ _ _ _ _ _ _ _ _ _ _ _ _ w386 w403 _ _ _ w441 _ _ _]
      tunnel: w317 -> [_ _ _ _ _ _ _ _ _ _ _ _ _ w385 w402 _ _ _ w440 _ _ _]
      event Timeout {
        n173 = event-data() -> ()  [unwired: 1 in, 2 out]
      }
      event "水样测试": Value Change {
        n174 = event-data() -> ()  [unwired: 1 in, 6 out]
        n175 = local write "启动测量模式"(T1."水样测试" ("启动测量模式")) -> ()
        n176 = call "CODCrMB_api.vi"("STEP"=enum16{"open", "read", "write", "close"}."write", "values"=u16[] [1], "starting address"=u16 4608) -> ()  [unwired: 6 in, 3 out]
      }
      event "标样核查": Value Change {
        n177 = event-data() -> ()  [unwired: 1 in, 6 out]
        n178 = local write "启动测量模式"(T1."标样核查" ("启动测量模式")) -> ()
        n179 = call "CODCrMB_api.vi"("STEP"=enum16{"open", "read", "write", "close"}."write", "values"=u16[] [2], "starting address"=u16 4608) -> ()  [unwired: 6 in, 3 out]
      }
      event "零点核查": Value Change {
        n180 = event-data() -> ()  [unwired: 1 in, 6 out]
        n181 = local write "启动测量模式"(T1."零点核查" ("启动测量模式")) -> ()
        n182 = call "CODCrMB_api.vi"("STEP"=enum16{"open", "read", "write", "close"}."write", "values"=u16[] [3], "starting address"=u16 4608) -> ()  [unwired: 6 in, 3 out]
      }
      event "跨度核查": Value Change {
        n183 = event-data() -> ()  [unwired: 1 in, 6 out]
        n184 = local write "启动测量模式"(T1."跨度核查" ("启动测量模式")) -> ()
        n185 = call "CODCrMB_api.vi"("STEP"=enum16{"open", "read", "write", "close"}."write", "values"=u16[] [4], "starting address"=u16 4608) -> ()  [unwired: 6 in, 3 out]
      }
      event "空白测试": Value Change {
        n186 = event-data() -> ()  [unwired: 1 in, 6 out]
        n187 = local write "启动测量模式"(T1."空白测试" ("启动测量模式")) -> ()
        n188 = call "CODCrMB_api.vi"("STEP"=enum16{"open", "read", "write", "close"}."write", "values"=u16[] [5], "starting address"=u16 4608) -> ()  [unwired: 6 in, 3 out]
      }
      event "平行样测试": Value Change {
        n189 = event-data() -> ()  [unwired: 1 in, 6 out]
        n190 = local write "启动测量模式"(T1."平行样测试" ("启动测量模式")) -> ()
        n191 = call "CODCrMB_api.vi"("STEP"=enum16{"open", "read", "write", "close"}."write", "values"=u16[] [6], "starting address"=u16 4608) -> ()  [unwired: 6 in, 3 out]
      }
      event "加标回收测试": Value Change {
        n192 = event-data() -> ()  [unwired: 1 in, 6 out]
        n193 = local write "启动测量模式"(T1."加标回收" ("启动测量模式")) -> ()
        n194 = call "CODCrMB_api.vi"("STEP"=enum16{"open", "read", "write", "close"}."write", "values"=u16[] [7], "starting address"=u16 4608) -> ()  [unwired: 6 in, 3 out]
      }
      event "空白校准": Value Change {
        n195 = event-data() -> ()  [unwired: 1 in, 6 out]
        n196 = local write "启动测量模式"(T1."空白校准" ("启动测量模式")) -> ()
        n197 = call "CODCrMB_api.vi"("STEP"=enum16{"open", "read", "write", "close"}."write", "values"=u16[] [8], "starting address"=u16 4608) -> ()  [unwired: 6 in, 3 out]
      }
      event "标样校准": Value Change {
        n198 = event-data() -> ()  [unwired: 1 in, 6 out]
        n199 = local write "启动测量模式"(T1."标样校准" ("启动测量模式")) -> ()
        n200 = call "CODCrMB_api.vi"("STEP"=enum16{"open", "read", "write", "close"}."write", "values"=u16[] [9], "starting address"=u16 4608) -> ()  [unwired: 6 in, 3 out]
      }
      event "停止": Value Change {
        n201 = event-data() -> ()  [unwired: 1 in, 6 out]
        n202 = Two Button Dialog(message="确认是否停止？" ("消息"), 1:"否" ("F按钮名称（“取消”）"), 2:"是" ("T按钮名称（“确定”）")) -> (T button?=w356:bool)
        n203 = case shown="真" w356 {
          frame False {
          }
          frame True {
            n204 = call "CODCrMB_api.vi"("STEP"=enum16{"open", "read", "write", "close"}."write", "values"=u16[] [12], "starting address"=u16 4608) -> ()  [unwired: 6 in, 3 out]
          }
        }
      }
      event "保存KB值": Value Change {
        n205 = event-data() -> ()  [unwired: 1 in, 6 out]
        n206 = local read "曲线斜率B"() -> (w367:sgl)
        n207 = local read "曲线斜率K"() -> (w368:sgl)
        n208 = Build Array(w368, w367) -> (w366:sgl[])
        n209 = call "FloatToHex.vi"("浮点数"=w366) -> ("DCBA整形输出"=w363:u16[])  [unwired: 10 in]
        n210 = call "CODCrMB_api.vi"("STEP"=enum16{"open", "read", "write", "close"}."write", "values"=w363, "starting address"=u16 4263) -> ()  [unwired: 6 in, 3 out]
      }
      event "定时启动": Value Change {
        n211 = event-data() -> ()  [unwired: 1 in, 6 out]
        n212 = flat-sequence {
          frame #0 {
            n213 = global read "CODcr全局变量.vi" "定时控制"() -> (w370:T7)
            n214 = call "周期设置.vi"("定时控制参数输入"=w370) -> ("定时控制参数输出"=w369:T7)  [unwired: 10 in]
            n215 = global write "CODcr全局变量.vi" "定时控制"(w369) -> ()
          }
          frame #1 {
            n216 = call <vilib>:"Application Directory.vi"() -> ("Application Directory"=w384:path)
            n217 = Build Path(base path=w384, name or relative path="data\\sys.ini" ("名称或相对路径")) -> (appended path=w382:path)
            n218 = call <vilib>:"Open Config Data.vi"("configuration file path"=w382) -> ("error out"=w378:errorcluster, "refnum"=w381:T10)  [unwired: 8 in, 1 out]
            n219 = vi-ref "CODCr库.lvlib:CODcr全局变量.vi"() -> (w380:refnum<vi>)
            n220 = call <userlib>:"Write Panel to INI__ogtk.vi"("error in (no error)"=w378, "VI ref"=w380, "refnum"=w381) -> ("error out"=w377:errorcluster, "refnum out"=w379:T10)  [unwired: 7 in]
            n221 = call <vilib>:"Close Config Data.vi"("error in (no error)"=w377, "refnum"=w379) -> ("error out"=w372:errorcluster, "file path"=w371:path)  [unwired: 8 in]
            n222 = Open/Create/Replace File(file path (use dialog)=w371, error in=w372) -> (refnum out=w375:refnum<file>, error out=w376:errorcluster)  [unwired: 4 in, 1 out]
            n223 = Flush File(refnum=w375, error in=w376) -> (refnum out=w374:refnum<file>, error out=w373:errorcluster)
            n224 = Close File(refnum=w374, error in=w373) -> ()  [unwired: 2 out]
          }
        }
      }
      event "打开串口": Value Change {
        n225 = event-data() -> ()  [unwired: 1 in, 6 out]
        n226 = global read "CODcr全局变量.vi" "VISA Resource"() -> (w393:refnum<visa-resource-name>)
        n227 = global read "CODcr全局变量.vi" "PORT"() -> (w387:string)
        n228 = global read "CODcr全局变量.vi" "IP"() -> (w388:string)
        n229 = call "串口配置.vi"("PORT"=w387, "IP"=w388, "请选择串口:"=w393) -> ("PORT 2"=w389:string, "IP 2"=w390:string, "确认 2"=w392:bool, "VISA资源名称 2"=w391:refnum<visa-resource-name>)  [unwired: 5 in]
        n230 = case shown="真" w392 {
          tunnel: w391 -> [_ w396]
          tunnel: w386 -> [_ w398]
          tunnel: w385 -> [_ w397]
          tunnel: w390 -> [_ w395]
          tunnel: w389 -> [_ w394]
          frame False {
          }
          frame True {
            n231 = global write "CODcr全局变量.vi" "VISA Resource"(w396) -> ()
            n232 = global write "CODcr全局变量.vi" "PORT"(w394) -> ()
            n233 = global write "CODcr全局变量.vi" "IP"(w395) -> ()
            n234 = Bundle By Name(cluster=cluster{"命令":string} {"命令"=""} ("元素"), "命令"="启用模块" ("名称（未命名）")) -> (w399:cluster{"命令":string})
            n235 = Enqueue Element(queue=w398, element=w399, error in (no error)=w397) -> ()  [unwired: 1 in, 3 out]
          }
        }
      }
      event "释放串口": Value Change {
        n236 = event-data() -> ()  [unwired: 1 in, 6 out]
        n237 = Two Button Dialog(message="确认是否释放串口，释放串口将导致通信失败！" ("消息")) -> (T button?=w404:bool)  [unwired: 2 in]
        n238 = case shown="真" w404 {
          tunnel: w403 -> [_ w407]
          tunnel: w402 -> [_ w406]
          frame False {
          }
          frame True {
            n239 = Bundle By Name(cluster=cluster{"命令":string} {"命令"=""} ("元素"), "命令"="停用模块" ("名称（未命名）")) -> (w408:cluster{"命令":string})
            n240 = Enqueue Element(queue=w407, element=w408, error in (no error)=w406) -> ()  [unwired: 1 in, 3 out]
          }
        }
      }
      event "MB通信方式选择": Value Change {
        n241 = event-data() -> ()  [unwired: 1 in, 6 out]
        n242 = flat-sequence {
          frame #0 {
            n243 = global write "CODcr全局变量.vi" "MB通信方式选择"("MB通信方式选择") -> ()
          }
          frame #1 {
            n244 = call <vilib>:"Application Directory.vi"() -> ("Application Directory"=w425:path)
            n245 = Build Path(base path=w425, name or relative path="data\\sys.ini" ("名称或相对路径")) -> (appended path=w423:path)
            n246 = call <vilib>:"Open Config Data.vi"("configuration file path"=w423) -> ("error out"=w419:errorcluster, "refnum"=w422:T10)  [unwired: 8 in, 1 out]
            n247 = vi-ref "CODCr库.lvlib:CODcr全局变量.vi"() -> (w421:refnum<vi>)
            n248 = call <userlib>:"Write Panel to INI__ogtk.vi"("error in (no error)"=w419, "VI ref"=w421, "refnum"=w422) -> ("error out"=w418:errorcluster, "refnum out"=w420:T10)  [unwired: 7 in]
            n249 = call <vilib>:"Close Config Data.vi"("error in (no error)"=w418, "refnum"=w420) -> ("error out"=w413:errorcluster, "file path"=w412:path)  [unwired: 8 in]
            n250 = Open/Create/Replace File(file path (use dialog)=w412, error in=w413) -> (refnum out=w416:refnum<file>, error out=w417:errorcluster)  [unwired: 4 in, 1 out]
            n251 = Flush File(refnum=w416, error in=w417) -> (refnum out=w415:refnum<file>, error out=w414:errorcluster)
            n252 = Close File(refnum=w415, error in=w414) -> ()  [unwired: 2 out]
          }
        }
      }
      event "写入消解温度时长": Value Change {
        n253 = event-data() -> ()  [unwired: 1 in, 6 out]
        n254 = local read "消解时长"() -> (w430:u16)
        n255 = local read "消解温度"() -> (w431:u16)
        n256 = Build Array(w431, w430) -> (w429:u16[])
        n257 = call "WordToHex.vi"("WORD"=w429) -> ("数组"=w426:u16[])  [unwired: 10 in]
        n258 = call "CODCrMB_api.vi"("STEP"=enum16{"open", "read", "write", "close"}."write", "values"=w426, "starting address"=u16 4257) -> ()  [unwired: 6 in, 3 out]
      }
      event "校时": Value Change {
        n259 = event-data() -> ()  [unwired: 1 in, 6 out]
        n260 = Get Date/Time In Seconds() -> (seconds since 1Jan1904=w439:timestamp)
        n261 = Build Array(w439) -> (w436:timestamp[])
        n262 = call "DateToHex.vi"("DATE"=w436) -> ("数组"=w435:u16[])  [unwired: 10 in]
        n263 = Insert Into Array(array=u16[] [13] ("values"), index=1 ("索引"), new element=w435) -> (w432:u16[])
        n264 = call "CODCrMB_api.vi"("STEP"=enum16{"open", "read", "write", "close"}."write", "values"=w432, "starting address"=u16 4608) -> ()  [unwired: 6 in, 3 out]
      }
      event "设置": Value Change {
        n265 = event-data() -> ()  [unwired: 1 in, 6 out]
        n266 = property on="窗格" class="Pane"("Origin"=T9 {"Horizontal"=0, "Vertical"=728} ("原点")) -> ()  [unwired: 2 in, 2 out]
        n267 = Bundle By Name(cluster=cluster{"命令":string} {"命令"=""} ("元素"), "命令"="CODCr读取参数" ("名称（未命名）")) -> (w442:cluster{"命令":string})
        n268 = Enqueue Element(queue=w441, element=w442, error in (no error)=w440) -> ()  [unwired: 1 in, 3 out]
      }
      event "返回": Value Change {
        w446 = FALSE ("可见")
        n269 = event-data() -> ()  [unwired: 1 in, 6 out]
        n270 = property on="窗格" class="Pane"("Origin"=T9 {"Horizontal"=0, "Vertical"=0} ("原点")) -> ()  [unwired: 2 in, 2 out]
        n271 = property on="写入消解温度时长" class="Bool"("Visible"=w446) -> ()  [unwired: 2 in, 2 out]
        n272 = property on="释放串口" class="Bool"("Visible"=w446) -> ()  [unwired: 2 in, 2 out]
        n273 = property on="打开串口" class="Bool"("Visible"=w446) -> ()  [unwired: 2 in, 2 out]
        n274 = property on="MB通信方式选择" class="Enum (严格)"("Visible"=w446) -> ()  [unwired: 2 in, 2 out]
      }
      event "曲线斜率K", "曲线斜率B", "消解温度", "消解时长": Mouse Down {
        n275 = event-data() -> ("CtlRef"=w450:refnum<vi>)  [unwired: 1 in, 7 out]
        n276 = property class="DigNum"(reference=w450) -> (reference out=w451:refnum<vi>, "Value"=w449:variant)  [unwired: 1 in, 1 out]
        n277 = Variant To Data(Variant=w449) -> (data=w448:sgl)  [unwired: 2 in, 1 out]
        n278 = call "CODCR数字键盘.vi"("OldNumber"=w448) -> ("NewNumber"=w452:sgl)
        n279 = property class="DigNum"(reference=w451, "Value"=w452) -> ()  [unwired: 1 in, 2 out]
      }
      event "隐藏按钮": Value Change {
        w453 = TRUE ("可见")
        n280 = event-data() -> ()  [unwired: 1 in, 6 out]
        n281 = property on="写入消解温度时长" class="Bool"("Visible"=w453) -> ()  [unwired: 2 in, 2 out]
        n282 = property on="释放串口" class="Bool"("Visible"=w453) -> ()  [unwired: 2 in, 2 out]
        n283 = property on="打开串口" class="Bool"("Visible"=w453) -> ()  [unwired: 2 in, 2 out]
        n284 = property on="MB通信方式选择" class="Enum (严格)"("Visible"=w453) -> ()  [unwired: 2 in, 2 out]
      }
    }
  }
  n285 = while {
    tunnel: w2 -> [w455]
    tunnel: w1 -> [w454]
    i -> [w463]
    stop <- FALSE stop-if-true
    n286 = First Call?() -> (First Call?: T/F=w458:bool)
    n287 = case shown="真" w458 {
      tunnel: w455 -> [w467 w472]
      tunnel: w454 -> [w466 w471]
      tunnel: [w467 w470] -> w457
      tunnel: [w466 w469] -> w456
      frame False {
      }
      frame True {
        n288 = Bundle By Name(cluster=cluster{"命令":string} {"命令"=""} ("元素"), "命令"="CODMn读取参数" ("名称（未命名）")) -> (w475:cluster{"命令":string})
        n289 = Enqueue Element(queue=w472, element=w475, timeout in ms (-1)=1000 ("超时毫秒(-1)"), error in (no error)=w471) -> (queue out=w470:refnum<queue>, error out=w469:errorcluster)  [unwired: 1 out]
      }
    }
    n290 = Get Queue Status(queue=w457, error in (no error)=w456) -> (queue out=w461:refnum<queue>, error out=w460:errorcluster, # elements in queue=w462:i32)  [unwired: 1 in, 5 out]
    n291 = Equal To 0?(x=w462) -> (x = 0?=w459:bool)
    n292 = case shown="真" w459 {
      tunnel: w461 -> [_ w477]
      tunnel: w460 -> [_ w476]
      frame False {
      }
      frame True {
        n293 = Bundle By Name(cluster=cluster{"命令":string} {"命令"=""} ("元素"), "命令"="CODCr读取" ("名称（未命名）")) -> (w479:cluster{"命令":string})
        n294 = Enqueue Element(queue=w477, element=w479, timeout in ms (-1)=1000 ("超时毫秒(-1)"), error in (no error)=w476) -> ()  [unwired: 3 out]
      }
    }
    n295 = Wait (ms)(milliseconds to wait=u32 1000 ("等待时间（毫秒）")) -> ()  [unwired: 1 out]
    "主循环次数" <- w463
  }
